vi "task2.4.vi"() -> ()   [LabVIEW 2021]
doc: "This example demonstrates how to continuously re-generate analog output data from a buffer in your computer's memory.\n\nRefer to your device documentation for pinouts and hardware capabilities."
uses:
  <vilib>/DAQmx/write.llb/DAQmx Write (Analog Wfm 1Chan NSamp).vi
  <vilib>/DAQmx/write.llb/DAQmx Write (Digital Bool 1Line 1Point).vi
  <vilib>/DAQmx/read.llb/DAQmx Read (Analog 1D Wfm NChan NSamp).vi
  <vilib>/DAQmx/create/channels.llb/DAQmx Create Channel (AO-Voltage-Basic).vi
  <vilib>/DAQmx/configure/timing.llb/DAQmx Timing (Sample Clock).vi
  <vilib>/DAQmx/create/channels.llb/DAQmx Create Channel (AI-Voltage-Basic).vi
  <vilib>/DAQmx/configure/trigger.llb/DAQmx Start Trigger (Digital Edge).vi
  <vilib>/DAQmx/miscellaneous.llb/DAQmx Fill In Error Info.vi
  <vilib>/DAQmx/create/channels.llb/DAQmx Create Channel (DO-Digital Output).vi
  <vilib>/measure/matone.llb/Extract Single Tone Information N Chan.vi
  <vilib>/Waveform/WDTFileIO.llb/ Write Waveform to File.vi
  <vilib>/Waveform/WDTFileIO.llb/ Write Waveforms to File (1D).vi
  <vilib>/express/express analysis/Spectral/Block/exnSpectralBlock spectral measurements peak poly.vi
  <vilib>/express/express analysis/Spectral/Block/exnSpectralBlock spectral measurements peak array WFM.vi
  <vilib>/express/express analysis/Spectral/Block/exnSpectralBlock spectral measurements peak WFM.vi
  <vilib>/express/express analysis/Spectral/XNode/ExpressSpectralMeasurementsBlockNode.xnode
  <vilib>/measure/NI_MABase.lvlib
  <vilib>/measure/NI_MAPro.lvlib
panel:
  out "Output Freq":cluster{"f0":dbl, "df":dbl, "magnitude":dbl[]}(graph)
  out "Input Freq":cluster{"f0":dbl, "df":dbl, "magnitude":dbl[]}[](graph)
  in  "Amplitude":dbl=1.0 format="%0.2p"
  in  "Frequency":dbl=10.0 format="%0.2p"
  in  "Waveform Type":u16(ring) items=["Sine Wave", "Triangle Wave", "Square Wave", "Sawtooth Wave"]
  in  "Input Channel 2":tag="Dev3/ai1"
  in  "Number of samples":i32=1000
  out "Input Voltage":waveform(dbl)[](graph)=[{"t0"=timestamp(3702416907.610318 s since 1904-01-01), "dt"=9.999999999999999e-05, "Y"=array[1000 elements], "attributes"=variant("NI_ChannelName"=variant(string "Dev6/ai0"), "NI_UnitDescription"=variant(string "Volts"))}, {"t0"=timestamp(3702416907.610332 s since 1904-01-01), "dt"=9.999999999999999e-05, "Y"=array[1000 elements], "attributes"=variant("NI_ChannelName"=variant(string "Dev6/ai1"), "NI_UnitDescription"=variant(string "Volts"))}]
  in  "Input Channel 1":tag="Dev3/ai0"
  in  "Min Input Voltage":dbl=-10.0
  in  "Max Input Voltage":dbl=10.0
  in  "Output sample rate":dbl=10000.0 format="%0.2f"
  out "Output Voltage":waveform(dbl)(graph)={"t0"=timestamp(0 s since 1904-01-01), "dt"=0.0001, "Y"=array[1000 elements]}
  in  "Max Voltage":dbl=10.0
  in  "Min Voltage":dbl=-10.0
  in  "Output Channel":tag="Dev3/ao0"
  # "Output Channel Settings"
  # "Output voltage"
  # "Input voltage"
  # "Input Channel Settings"
  # "Waveform Settings"
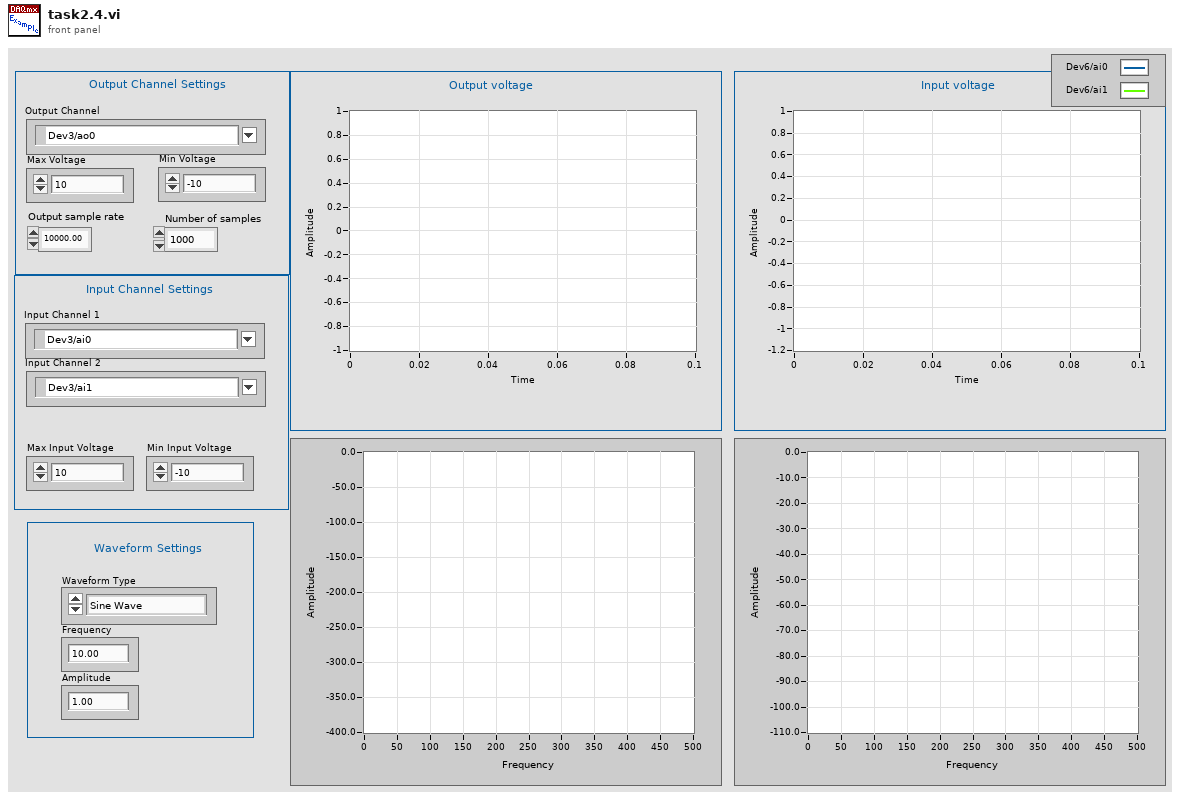
[diagram p1: front panel]
types:
  T1 = cluster{"Output sample rate":dbl, "Number of samples":i32}
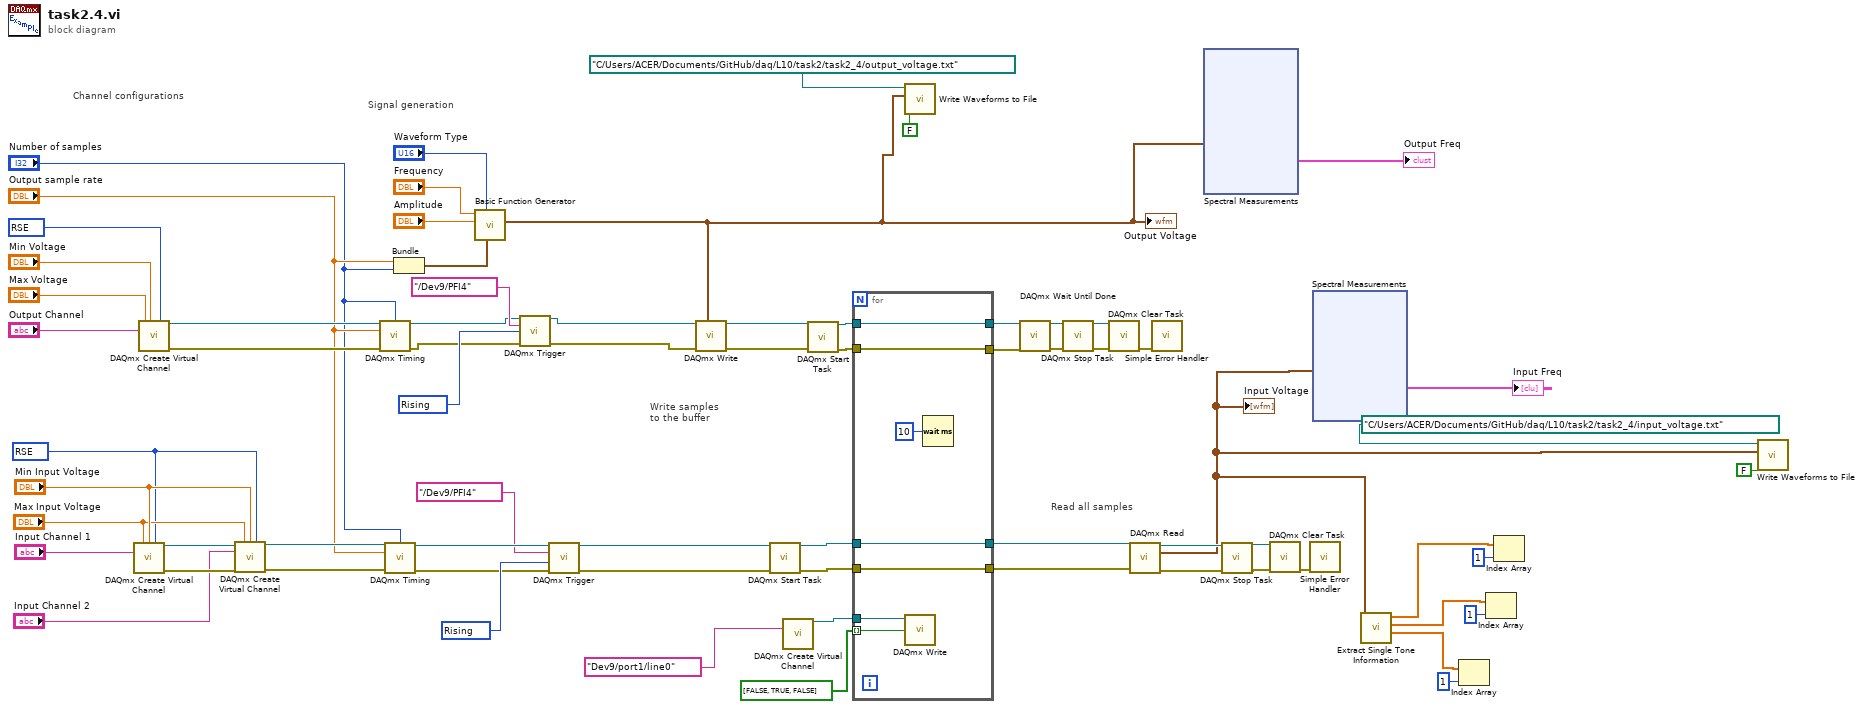
[diagram p0: block diagram]
diagram:
  w17 = 10280 items=["Rising"=10280, "Falling"=10171] ("edge")
  w21 = 10280 items=["Rising"=10280, "Falling"=10171] ("edge")
  w45 = 10083 items=["Default"=-1, "RSE"=10083, "NRSE"=10078, "Differential"=10106, "Pseudodifferential"=12529] ("input terminal configuration")
  w59 = 10083 items=["Default"=-1, "RSE"=10083, "NRSE"=10078, "Differential"=10106, "Pseudodifferential"=12529] ("input terminal configuration")
  # "Read all samples"
  # "Write samples\nto the buffer"
  # "Signal generation"
  # "Channel configurations"
  n1 = call-poly <vilib>:"DAQmx Create Virtual Channel.vi"("maximum value"="Max Input Voltage", "minimum value"="Min Input Voltage", "input terminal configuration"=w45, "physical channels"="Input Channel 1") -> ("task out"=w55:refnum<k21>, "error out"=w56:errorcluster)  [unwired: 10 in]
  n2 = call-poly <vilib>:"DAQmx Create Virtual Channel.vi"("maximum value"="Max Voltage", "minimum value"="Min Voltage", "output terminal configuration"=w59, "physical channels"="Output Channel") -> ("task out"=w63:refnum<k21>, "error out"=w64:errorcluster)  [unwired: 10 in]
  n3 = call-poly <vilib>:"DAQmx Create Virtual Channel.vi"("task in"=w55, "maximum value"="Max Input Voltage", "minimum value"="Min Input Voltage", "input terminal configuration"=w45, "physical channels"="Input Channel 2", "error in"=w56) -> ("task out"=w54:refnum<k21>, "error out"=w53:errorcluster)  [unwired: 8 in]
  n4 = call-poly <vilib>:"DAQmx Timing.vi"("task/channels in"=w63, "samples per channel"="Number of samples", "rate"="Output sample rate", "error in"=w64) -> ("task out"=w22:refnum<k21>, "error out"=w20:errorcluster)  [unwired: 10 in]
  n5 = call-poly <vilib>:"DAQmx Timing.vi"("task/channels in"=w54, "samples per channel"="Number of samples", "rate"="Output sample rate", "error in"=w53) -> ("task out"=w14:refnum<k21>, "error out"=w16:errorcluster)  [unwired: 10 in]
  n6 = Bundle "Bundle"("Output sample rate"="Output sample rate", "Number of samples"="Number of samples") -> (w44:T1)  [unwired: 1 in]
  n7 = call <vilib>:"Basic Function Generator.vi"("sampling info"=w44, "signal type"="Waveform Type", "amplitude"="Amplitude", "frequency"="Frequency") -> ("signal out"=w8:waveform(dbl))  [unwired: 5 in, 2 out]
  "Output Voltage" <- w8
  n8 = call-poly <vilib>:"DAQmx Trigger.vi"("task/channels in"=w22, "source"=tag "/Dev9/PFI4", "edge"=w21, "error in"=w20) -> ("task out"=w25:refnum<k21>, "error out"=w24:errorcluster)  [unwired: 10 in]
  n9 = call-poly <vilib>:"DAQmx Trigger.vi"("task/channels in"=w14, "source"=tag "/Dev9/PFI4", "edge"=w17, "error in"=w16) -> ("task out"=w19:refnum<k21>, "error out"=w18:errorcluster)  [unwired: 10 in]
  n10 = call-poly <vilib>:"DAQmx Write.vi"("task/channels in"=w25, "data"=w8, "error in"=w24) -> ("task out"=w27:refnum<k21>, "error out"=w26:errorcluster)  [unwired: 10 in, 1 out]
  n11 = call <vilib>:"DAQmx Start Task.vi"("task/channels in"=w19, "error in"=w18) -> ("task out"=w34:refnum<k21>, "error out"=w35:errorcluster)  [unwired: 12 in]
  n12 = call-poly <vilib>:"DAQmx Create Virtual Channel.vi"("lines"=tag "Dev9/port1/line0") -> ("task out"=w32:refnum<k21>)  [unwired: 13 in, 1 out]
  n13 = call <vilib>:"DAQmx Start Task.vi"("task/channels in"=w27, "error in"=w26) -> ("task out"=w36:refnum<k21>, "error out"=w37:errorcluster)  [unwired: 12 in]
  n14 = for {
    tunnel: bool[] [FALSE, TRUE, FALSE] -> [w76] mode=indexing
    tunnel: w35 -> [w72]
    tunnel: w34 -> [w73]
    tunnel: w37 -> [w74]
    tunnel: w36 -> [w75]
    tunnel: [w75] -> w31
    tunnel: [w74] -> w30
    tunnel: [w73] -> w29
    tunnel: [w72] -> w28
    tunnel: w32 -> [w71]
    n15 = call-poly <vilib>:"DAQmx Write.vi"("task/channels in"=w71, "data"=w76) -> ()  [unwired: 11 in, 3 out]
    n16 = Wait (ms)(milliseconds to wait=u32 10) -> ()  [unwired: 1 out]
  }
  n17 = call-poly <vilib>:"Write Waveforms to File.vi"("append to file? (new file:F)"=FALSE, "waveform"=w8, "file path (dialog if empty)"=path "C:/Users/ACER/Documents/GitHub/daq/L10/task2/task2_4/output_voltage.txt") -> ()  [unwired: 7 in, 2 out]
  n18 = call <vilib>:"DAQmx Wait Until Done.vi"("task/channels in"=w31, "error in"=w30) -> ("task out"=w41:refnum<k21>, "error out"=w40:errorcluster)  [unwired: 12 in]
  n19 = call <vilib>:"DAQmx Stop Task.vi"("task/channels in"=w41, "error in"=w40) -> ("task out"=w66:refnum<k21>, "error out"=w65:errorcluster)  [unwired: 12 in]
  n20 = call <vilib>:"DAQmx Clear Task.vi"("task in"=w66, "error in"=w65) -> ("error out"=w70:errorcluster)  [unwired: 13 in]
  n21 = call-poly <vilib>:"DAQmx Read.vi"("task/channels in"=w29, "error in"=w28) -> ("task out"=w57:refnum<k21>, "data"=w1:waveform(dbl)[], "error out"=w58:errorcluster)  [unwired: 11 in]
  "Input Voltage" <- w1
  n22 = call <vilib>:"Simple Error Handler.vi"("error in (no error)"=w70) -> ()  [unwired: 4 in, 5 out]
  n23 = xnode "Spectral Measurements"("Signals"=w8) -> ("FFT - (Peak)"=→"Output Freq":cluster{"f0":dbl, "df":dbl, "magnitude":dbl[]})  [unwired: 1 in, 2 out]
  n24 = call <vilib>:"DAQmx Stop Task.vi"("task/channels in"=w57, "error in"=w58) -> ("task out"=w61:refnum<k21>, "error out"=w62:errorcluster)  [unwired: 12 in]
  n25 = call <vilib>:"DAQmx Clear Task.vi"("task in"=w61, "error in"=w62) -> ("error out"=w60:errorcluster)  [unwired: 13 in]
  n26 = call <vilib>:"Simple Error Handler.vi"("error in (no error)"=w60) -> ()  [unwired: 4 in, 5 out]
  n27 = xnode "Spectral Measurements"("Signals"=w1) -> ("FFT - (Peak)"=→"Input Freq":cluster{"f0":dbl, "df":dbl, "magnitude":dbl[]}[])  [unwired: 1 in, 2 out]
  n28 = call-poly <vilib>:"Extract Single Tone Information.vi"("time signals in"=w1) -> ("detected phases (deg)"=w6:dbl[], "detected amplitudes"=w7:dbl[], "detected frequencies"=w2:dbl[])  [unwired: 5 in, 3 out]
  n29 = Index Array(array=w6, index=1) -> ()  [unwired: 1 out]
  n30 = Index Array(array=w7, index=1) -> ()  [unwired: 1 out]
  n31 = Index Array(array=w2, index=1) -> ()  [unwired: 1 out]
  n32 = call-poly <vilib>:"Write Waveforms to File.vi"("append to file? (new file:F)"=FALSE, "waveform array"=w1, "file path (dialog if empty)"=path "C:/Users/ACER/Documents/GitHub/daq/L10/task2/task2_4/input_voltage.txt") -> ()  [unwired: 7 in, 2 out]
